vi "Wait For Previous.vi"(8 "error in (no error)":errorcluster, 9 "timeout in ms (0)":i32 format="%d ms", 11 "Transfer Group in":refnum<class "Transfer Group.lvclass">) -> (0 "error out":errorcluster, 1 "first iteration":bool, 2 "ready for next":bool, 3 "Transfer Group out":refnum<class "Transfer Group.lvclass">)   [LabVIEW 2017, in "DSF Core.lvlib" / "Transfer Group.lvclass"]
uses:
  Transfer Group.lvclass
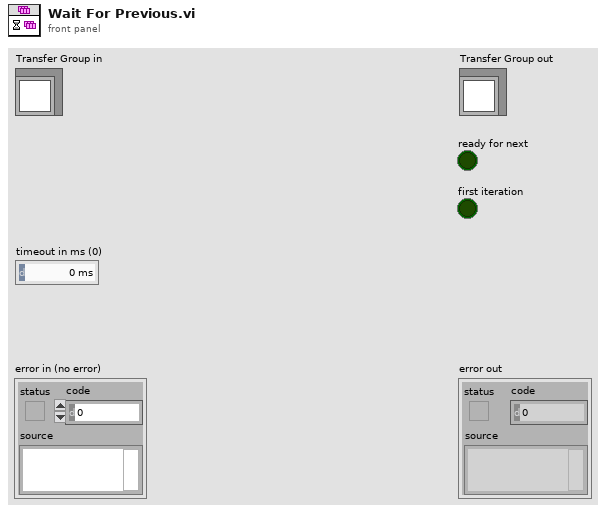
[diagram p1: front panel]
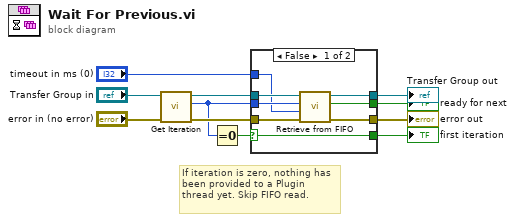
[diagram p0: block diagram]
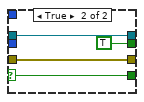
[diagram p2: hidden frame]
diagram:
  # "If iteration is zero, nothing has been provided to a Plugin thread yet. Skip FIFO read."
  n1 = call "Get Iteration.vi"("error in (no error)"="error in (no error)", "Transfer Group in"="Transfer Group in") -> ("error out"=w10:errorcluster, "iteration"=w9:u64, "Transfer Group out"=w8:refnum<class "Transfer Group.lvclass">)  [unwired: 7 in]
  n2 = Equal To 0?(x=w9) -> (x = 0?=w11:bool)
  n3 = case shown="False" w11 {
    selector: w11 -> [w12 w20]
    tunnel: w10 -> [w19 w23]
    tunnel: [w18 w22] -> w6
    tunnel: [w17 w23] -> w5
    tunnel: w8 -> [w16 w22]
    tunnel: w9 -> [w15 _]
    tunnel: [w13 TRUE ("iteration valid?")] -> w3
    tunnel: "timeout in ms (0)" -> [w14 _]
    tunnel: [w12 w20] -> w1
    frame False {
      n4 = call "Retrieve from FIFO.vi"("error in (no error)"=w19, "timeout in ms (0)"=w14, "expected iteration"=w15, "Transfer Group in"=w16) -> ("error out"=w17:errorcluster, "ready"=w13:bool, "Transfer Group out"=w18:refnum<class "Transfer Group.lvclass">)  [unwired: 5 in]
    }
    frame True {
    }
  }
  "error out" <- w5
  "Transfer Group out" <- w6
  "ready for next" <- w3
  "first iteration" <- w1
